vi "Configurazione strumenti.vi"() -> ()   [LabVIEW 2012]
panel:
  out "Beep":string
  out "Versione strumento":string
  out "Tipo di strumento":string
  out "Tensione":string
  in  "adr":string="4"
  out "tensione":dbl
  out "message":string=" INSTRUCTIONS:\r\rNormal Use:  When using subVIs that incorporate the error in/error out (or error I/O) structure, place this handler where you want to inform the user of an error, typically at the end of the I/O data path, as the last action of the program.  If the error in error? is ERROR, the handler creates a message describing the error and its source.  If the type of dialog = 1 (default), the message is displayed to the user, who can only acknowedge it.  If the type = 2, the user can acknowledge the message or abort execution; aborting a program with active I/O is not recommended.  If the type = 0, no message is displayed; this is used to process the error programmatically, and the error out cluster elements are wired to individual terminals for that reason.  \r\rOther Use:\n\r\nlocal testing.  To test the error code of a subVI or function that does not have the error I/O structure, you can wire its error code and a source string to the local error code and error source inputs.  If error in error? indicates no error and error code is not equal to 0, the local code and source are substituted for the error in values, and error? is set TRUE (ERROR)."
  out "error out":errorcluster
  out "Stringa":string
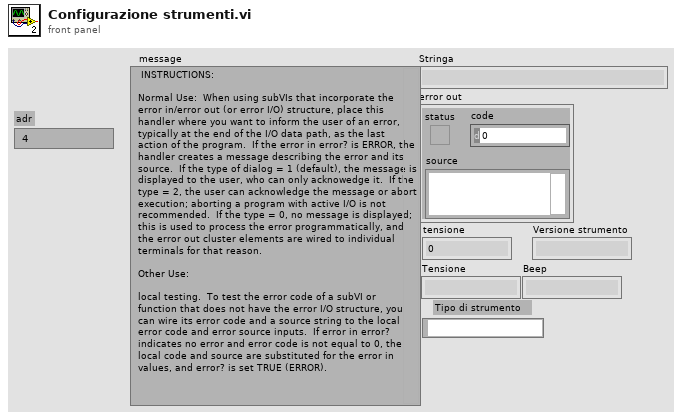
[diagram p1: front panel]
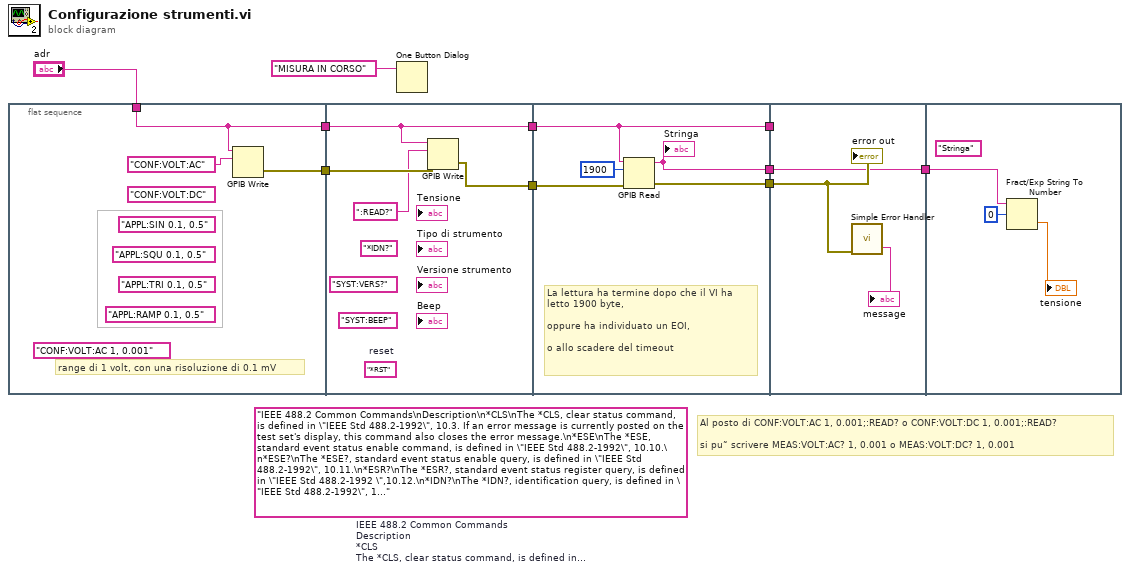
[diagram p0: block diagram]
diagram:
  (unwired) "IEEE 488.2 Common Commands\nDescription\n*CLS\nThe *CLS, clear status command, is defined in \"IEEE Std 488.2-1992\", 10.3. If an error message is currently posted on the test set's display, this command also closes the error message.\n*ESE\nThe *ESE, standard event status enable command, is defined in \"IEEE Std 488.2-1992\", 10.10.\n*ESE?\nThe *ESE?, standard event status enable query, is defined in \"IEEE Std 488.2-1992\", 10.11.\n*ESR?\nThe *ESR?, standard event status register query, is defined in \"IEEE Std 488.2-1992 \",10.12.\n*IDN?\nThe *IDN?, identification query, is defined in \"IEEE Std 488.2-1992\", 10.14.*IDN? is used to retrieve information about the test set in ASCII format.\n*IDN?, returns ASCII codes 32 through 126 excluding comma and semicolon in four comma separated fields. Field 1 returns the manufacturer, field 2 returns the instrument model number, field 3 returns the serial number, field 4 returns 0.\n*OPC\nThe *OPC, operation complete command, is defined in \"IEEE 488.2-1992\", 10.18. *OPC causes the test set to continuously sense the No Operation Pending flag. When the No Operation Pending flag becomes TRUE, the OPC event bit in the standard event status register (ESR) is set to indicate that the state of all pending operations is completed. The *OPC common command is not recommended for use as an overlapped command.\n*OPC?\nThe *OPC?, operation complete query, is defined in \"IEEE Std 488.2-1992\", 10.19. The *OPC? query allows synchronization between the controller and the test set using either the message available (MAV) bit in the status byte, or a read of the output OPC?. The *OPC? query does not effect the OPC event bit in the Standard Event Status Register (ESR). The *OPC? common command is not recommended for use as an overlapped command.\n*OPT?\nThe *OPT?, option identification query, is defined in \"IEEE Std 488.2-1992\", 10.20. Each option will have a unique name, that name will be retuned with the query.\n*RST\nThe *RST, full preset command, is defined in \"IEEE Std 488.2-1992\", 10.32. *RST is the recommended command when performing a full preset on the test set. A *RST restores the majority of settings to their default values.\n\t¥\t*RST sets trigger arm to single\n\t¥\tPRESet2 sets trigger arm to continuous\n*SRE\nThe *SRE, service request enable command, is defined in \"IEEE Std 488.2-1992\", 10.34. The parameter range for this command is 0 through 255.\n*SRE?\nThe *SRE?, service request enable query, is defined in \"IEEE Std 488.2-1992\", 10.35. Values returned by this query range from 0 through 255.\n*STB?\nThe *STB?, read status byte query, is defined in \"IEEE Std 488.2-1992\", 10.36. Values returned by this query range from 0 through 255.\n*TST?\nThe test set's implementation of *TST? does not follow the \"IEEE Std 488.2-1992\" section 10.38 definition. Rather, the test set's implementation is as described in the \"Verifying the Test Set\" (Self Test) topic in the Related Topics below. Values returned by this query are 0 (pass) and -330 (fail).\n*WAI\nThe *WAI, wait-to-continue command, is defined in \"IEEE Std 488.2-1992\", 10.39. The *WAI command prevents the test set from executing any further commands or queries until all pending operation flags are false. The *WAI common command is not recommended for use as an overlapped command."  # IEEE 488.2 Common Commands Description *CLS The *CLS, clear status command, is defined in "IEEE Std 488.2-1992", 10.3. If an error message is currently posted on the test set's display, this command also closes the error message. *ESE The *ESE, standard event status enable command, is defined in "IEEE Std 488.2-1992", 10.10. *ESE? The *ESE?, standard event status enable query, is defined in "IEEE Std 488.2-1992", 10.11. *ESR? The *ESR?, standard event status register query, is defined in "IEEE Std 488.2-1992 ",10.12. *IDN? The *IDN?, identification query, is defined in "IEEE Std 488.2-1992", 10.14.*IDN? is used to retrieve information about the test set in ASCII format. *IDN?, returns ASCII codes 32 through 126 excluding comma and semicolon in four comma separated fields. Field 1 returns the manufacturer, field 2 returns the instrument model number, field 3 returns the serial number, field 4 returns 0. *OPC The *OPC, operation complete command, is defined in "IEEE 488.2-1992", 10.18. *OPC causes the test set to continuously sense the No Operation Pending flag. When the No Operation Pending flag becomes TRUE, the OPC event bit in the standard event status register (ESR) is set to indicate that the state of all pending operations is completed. The *OPC common command is not recommended for use as an overlapped command. *OPC? The *OPC?, operation complete query, is defined in "IEEE Std 488.2-1992", 10.19. The *OPC? query allows synchronization between the controller and the test set using either the message available (MAV) bit in the status byte, or a read of the output OPC?. The *OPC? query does not effect the OPC event bit in the Standard Event Status Register (ESR). The *OPC? common command is not recommended for use as an overlapped command. *OPT? The *OPT?, option identification query, is defined in "IEEE Std 488.2-1992", 10.20. Each option will have a unique name, that name will be retuned with the query. *RST The *RST, full preset command, is defined in "IEEE Std 488.2-1992", 10.32. *RST is the recommended command when performing a full preset on the test set. A *RST restores the majority of settings to their default values. 	¥	*RST sets trigger arm to single 	¥	PRESet2 sets trigger arm to continuous *SRE The *SRE, service request enable command, is defined in "IEEE Std 488.2-1992", 10.34. The parameter range for this command is 0 through 255. *SRE? The *SRE?, service request enable query, is defined in "IEEE Std 488.2-1992", 10.35. Values returned by this query range from 0 through 255. *STB? The *STB?, read status byte query, is defined in "IEEE Std 488.2-1992", 10.36. Values returned by this query range from 0 through 255. *TST? The test set's implementation of *TST? does not follow the "IEEE Std 488.2-1992" section 10.38 definition. Rather, the test set's implementation is as described in the "Verifying the Test Set" (Self Test) topic in the Related Topics below. Values returned by this query are 0 (pass) and -330 (fail). *WAI The *WAI, wait-to-continue command, is defined in "IEEE Std 488.2-1992", 10.39. The *WAI command prevents the test set from executing any further commands or queries until all pending operation flags are false. The *WAI common command is not recommended for use as an overlapped command.
  # "Al posto di CONF:VOLT:AC 1, 0.001;:READ? o CONF:VOLT:DC 1, 0.001;:READ?\n\nsi pu˜ scrivere MEAS:VOLT:AC? 1, 0.001 o MEAS:VOLT:DC? 1, 0.001"
  n1 = flat-sequence {
    tunnel: [w12] -> w10
    tunnel: [w13] -> w8
    tunnel: "adr" -> [w12]
    tunnel: w10 -> [w17]
    tunnel: [w17] -> w9
    tunnel: w8 -> [w16]
    tunnel: [w15] -> w6
    tunnel: w9 -> [w22]
    tunnel: [w22] -> w7
    tunnel: w6 -> [w21]
    tunnel: [w20] -> w5
    tunnel: [w18] -> w1
    tunnel: w7 -> [_]
    tunnel: w5 -> [w24]
    tunnel: [w23] -> w2
    tunnel: w1 -> [w23]
    tunnel: w2 -> [w27]
    frame #0 {
      (unwired) "APPL:RAMP 0.1, 0.5" ("data")
      (unwired) "APPL:TRI 0.1, 0.5" ("data")
      (unwired) "APPL:SQU 0.1, 0.5" ("data")
      (unwired) "APPL:SIN 0.1, 0.5" ("data")
      (unwired) "CONF:VOLT:AC 1, 0.001" ("data")
      (unwired) "CONF:VOLT:DC" ("reset")
      # "range di 1 volt, con una risoluzione di 0.1 mV"
      n2 = GPIB Write(0:w12, 1:"CONF:VOLT:AC") -> (6:w13:errorcluster)  [unwired: 3 in, 1 out]
    }
    frame #1 {
      (unwired) "*RST"  # reset
      (unwired) "SYST:BEEP"
      (unwired) "SYST:VERS?" ("data")
      (unwired) "*IDN?" ("data")
      n3 = GPIB Write(0:w17, 1:":READ?", 3:w16) -> (6:w15:errorcluster)  [unwired: 2 in, 1 out]
    }
    frame #2 {
      # "La lettura ha termine dopo che il VI ha letto 1900 byte,\n\noppure ha individuato un EOI,\n\no allo scadere del timeout"
      n4 = GPIB Read(0:w22, 1:1900 ("byte count"), 3:w21) -> (5:w18:string, 7:w20:errorcluster)  [unwired: 2 in, 1 out]
      "Stringa" <- w18
    }
    frame #3 {
      n5 = call <vilib>:"Simple Error Handler.vi"("error in (no error)"=w24) -> ("message"=→"message":string)  [unwired: 4 in, 4 out]
      "error out" <- w24
    }
    frame #4 {
      (unwired) "Stringa"
      n6 = Fract/Exp String To Number(string=w27, offset=0) -> (number=→"tensione":dbl)  [unwired: 2 in, 1 out]
    }
  }
  n7 = One Button Dialog(message="MISURA IN CORSO") -> ()  [unwired: 1 in, 1 out]
